vi "Read IED Setpoint Status.vi"(11 "IED Setpoint Status Msg in":refnum<class "IED Setpoint Status Msg.lvclass">) -> (0 "Error String":string, 1 "Variable Name":string, 2 "IED Name":string, 3 "IED Setpoint Status Msg out":refnum<class "IED Setpoint Status Msg.lvclass">, 4 "Status":T1)   [LabVIEW 2015, in "SCADA Core.lvlib" / "IED Setpoint Status Msg.lvclass"]
uses:
  IED Setpoint Status Msg.lvclass
  IED Setpoint Status.ctl
  IED Setpoint Status Msg.lvclass/IED Setpoint Status Msg.ctl
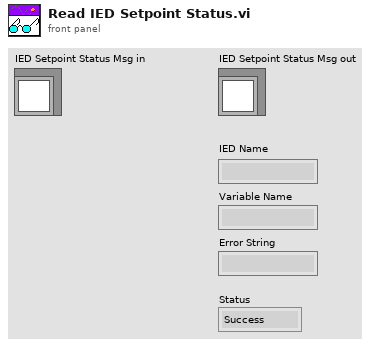
[diagram p1: front panel]
types:
  T1 = typedef "SCADA Core.lvlib/IED Setpoint Status Msg.lvclass/IED Setpoint Status.ctl" = enum16{"Success", "Failure", "Multiple Success", "Multiple Failure"}
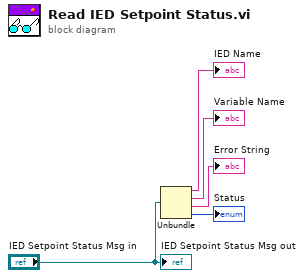
[diagram p0: block diagram]
diagram:
  n1 = Unbundle("IED Setpoint Status Msg in") -> (→"IED Name":string, →"Variable Name":string, →"Error String":string, →"Status":T1)
  "IED Setpoint Status Msg out" <- "IED Setpoint Status Msg in"
